vi "Fit Peaks.vi"(8 "error in (no error)":errorcluster, 10 "Y":dbl[](array[numeric]), 11 "Ocean Optics Driver in":refnum<class "Ocean Optics Driver.lvclass">) -> (0 "error out":errorcluster, 3 "Ocean Optics Driver out":refnum<class "Ocean Optics Driver.lvclass">)   [LabVIEW 2016, in "Ocean Optics Driver.lvclass"]
uses:
  Ocean Optics Driver.lvclass
  C:/github/NHMFL_Core/Libraries/Instruments/Spectrometer Driver/Spectrometer Driver.lvclass
  Spectrometer Driver/Spectrometer Driver.lvclass/Spectrometer Driver.ctl
  Ocean Optics Driver.lvclass/Ocean Optics Driver.ctl
  Spectrometer Driver/Read Wavelengths.vi
  Spectrometer Driver/Write Peaks.vi
  Read Ocean optics configuration.vi
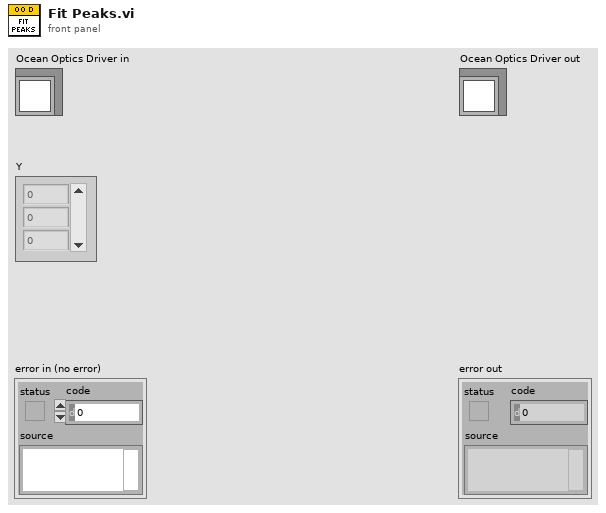
[diagram p1: front panel]
types:
  T1 = typedef "Ocean optics configuration.ctl" = cluster{"Integration time":dbl, "Fit parameters":T2, "Fit":bool, "Auto-update params":bool, "Window width":dbl, "Save spectra":bool}
  T2 = typedef "Multi-peak Parameters.ctl" = cluster{"Peaks":T3[], "Slope":dbl, "Intercept":dbl, "Function":enum16{"Gauss", "Lorentz"}, "Repeat fit":i32}
  T3 = typedef "Peak Parameters.ctl" = cluster{"Amplitude":dbl, "Center":dbl, "Width":dbl}
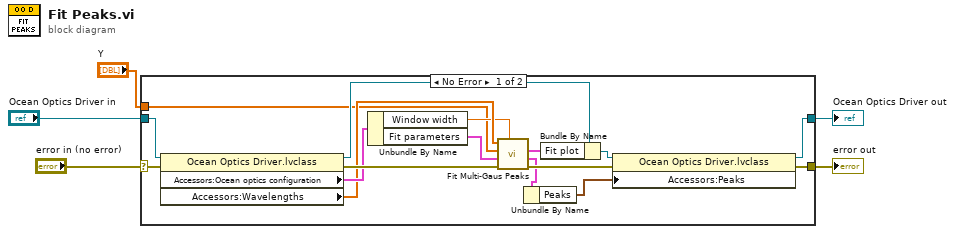
[diagram p0: block diagram]
diagram:
  n1 = case shown="No Error" "error in (no error)" {
    selector: "error in (no error)" -> [w21 w23]
    tunnel: [w10 w23] -> w4
    tunnel: [w8 w22] -> w2
    tunnel: "Ocean Optics Driver in" -> [w20 w22]
    tunnel: "Y" -> [w13 _]
    frame No Error {
      n2 = property class="Ocean Optics Driver.lvclass"(reference=w20, error in=w21) -> (reference out=w19:refnum<class "Ocean Optics Driver.lvclass">, error out=w18:errorcluster, "Accessors:Ocean optics configuration"=w17:T1, "Accessors:Wavelengths"=w15:dbl[])
      n3 = Unbundle By Name(w17) -> ("Window width"=w14:dbl, "Fit parameters"=w16:T2)
      n4 = call "Fit Multi-Gaus Peaks.vi"("Window width"=w14, "Error In"=w18, "Fit parameters"=w16, "Y"=w13, "X"=w15) -> ("Error Out"=w12:errorcluster, "Fit parameters out"=w7:T2, "Fit plot"=w11:cluster{"Array":dbl[], "Array":dbl[]})  [unwired: 4 in]
      n5 = Unbundle By Name(w7) -> ("Peaks"=w6:T3[])
      n6 = Bundle By Name(cluster=w19, "Fit plot"=w11) -> (w9:refnum<class "Ocean Optics Driver.lvclass">)
      n7 = property class="Ocean Optics Driver.lvclass"(reference=w9, error in=w12, "Accessors:Peaks"=w6) -> (reference out=w8:refnum<class "Ocean Optics Driver.lvclass">, error out=w10:errorcluster)
    }
    frame Error {
    }
  }
  "error out" <- w4
  "Ocean Optics Driver out" <- w2
